vi "Write LCR Meter.lvclass.vi"(10 "LCR Meter.lvclass":refnum<class "LCR Meter.lvclass">, 11 "LCR-Measurement in":refnum<class "LCR-Meas.lvclass">) -> (3 "LCR-Measurement out":refnum<class "LCR-Meas.lvclass">)   [LabVIEW 2020, in "LCR-Meas.lvclass"]
uses:
  LCR-Meas.lvclass
  Instruments/LCR Meter/LCR Meter.lvclass
  LCR-Meas.lvclass/LCR-Meas.ctl
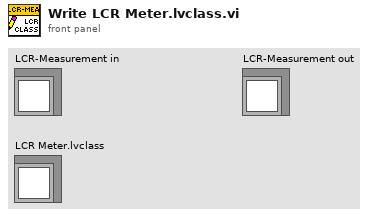
[diagram p1: front panel]
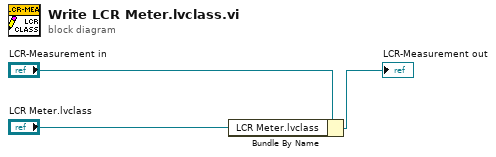
[diagram p0: block diagram]
diagram:
  n1 = Bundle By Name(cluster="LCR-Measurement in", "LCR Meter.lvclass"="LCR Meter.lvclass") -> (→"LCR-Measurement out":refnum<class "LCR-Meas.lvclass">)
